vi "String To Number(I64)_csm.vi"(5 "String":string) -> (0 "Numeric(I64)":u64)   [LabVIEW 2017, in "API String Arguments Support.lvlib"]
uses:
  API String Arguments Support.lvlib
  35e04dae-fb20-45f2-b6e6-a1e99b0bae27.vi
  c7c8f582-3164-4c23-83d8-8f64db7f198b.vi
  <userlib>/_NEVSTOP/Communicable State Machine(CSM)/Communicable State Machine.lvlib
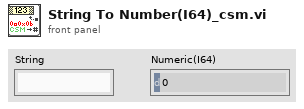
[diagram p1: front panel]
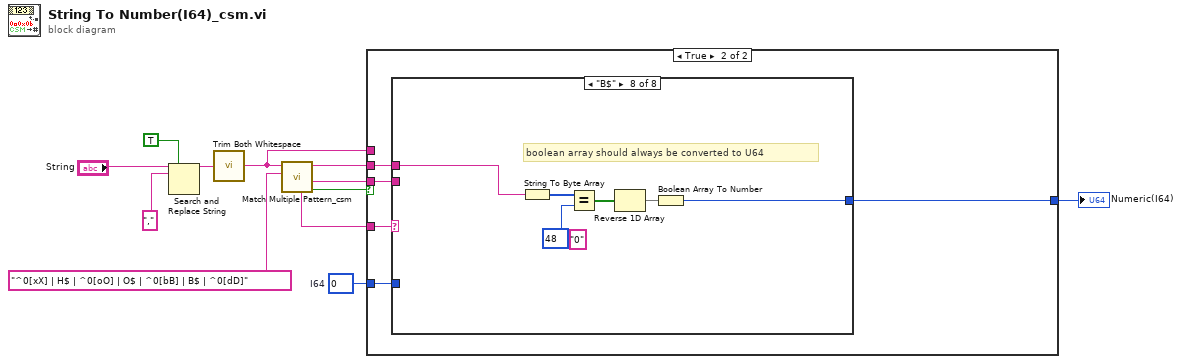
[diagram p0: block diagram]
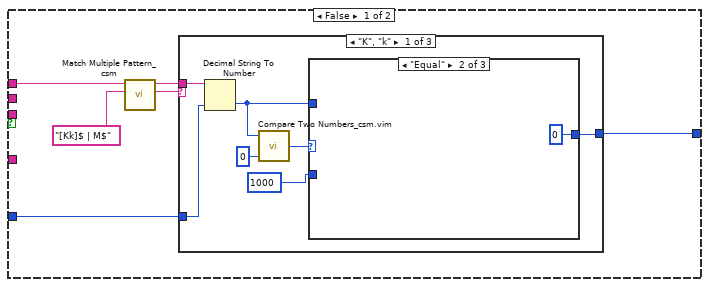
[diagram p2: hidden frame]
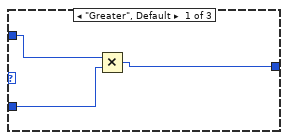
[diagram p3: hidden frame]
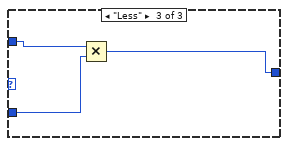
[diagram p4: hidden frame]
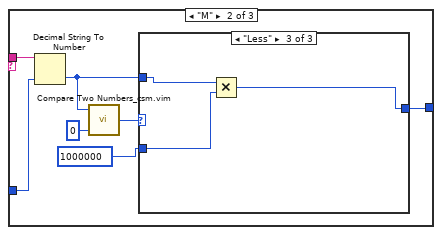
[diagram p5: hidden frame]
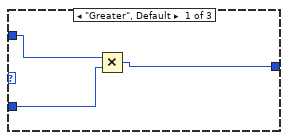
[diagram p6: hidden frame]
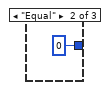
[diagram p7: hidden frame]
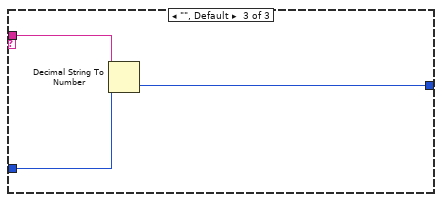
[diagram p8: hidden frame]
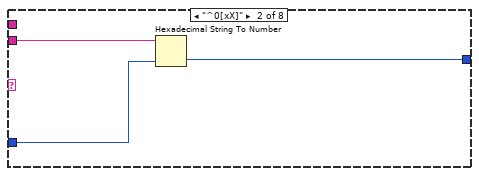
[diagram p10: hidden frame]
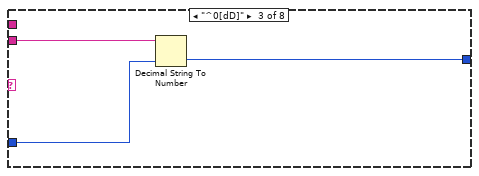
[diagram p11: hidden frame]
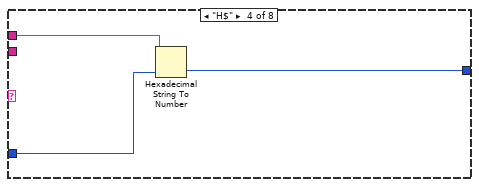
[diagram p12: hidden frame]
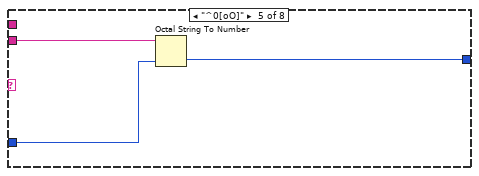
[diagram p13: hidden frame]
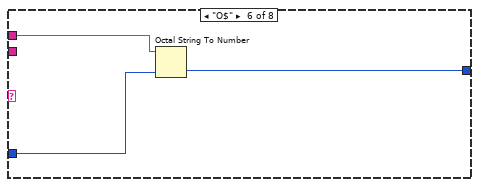
[diagram p14: hidden frame]
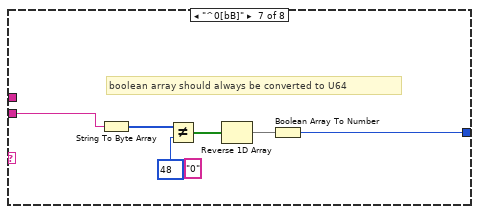
[diagram p15: hidden frame]
diagram:
  w1 = i64 0  # I64
  n1 = Search and Replace String(replace all?=TRUE ("replace all? (F)"), input string="String", search string=",") -> (result string=w9:string)  [unwired: 5 in, 3 out]
  n2 = call <userlib>:"Trim Both Whitespace.vi"("string"=w9) -> ("trimmed string"=w2:string)  [unwired: 1 in]
  n3 = call "Match Multiple Pattern_csm.vi"("regular expression"="^0[xX] | H$ | ^0[oO] | O$ | ^0[bB] | B$ | ^0[dD]", "string"=w2) -> ("Found?"=w7:bool, "after substring"=w5:string, "before substring"=w4:string, "pattern matched"=w6:string)  [unwired: 5 in, 1 out]
  n4 = case shown="True" w7 {
    tunnel: w6 -> [_ w54]
    tunnel: w5 -> [_ w53]
    tunnel: w4 -> [_ w52]
    tunnel: [w13 w51] -> w3
    tunnel: w2 -> [w14 _]
    tunnel: w1 -> [w15 w50]
    frame False {
      n5 = call "Match Multiple Pattern_csm.vi"("regular expression"="[Kk]$ | M$", "string"=w14) -> ("match substring"=w17:string, "before substring"=w16:string)  [unwired: 5 in, 3 out]
      n6 = case shown="\"K\", \"k\"" w17 {
        tunnel: [w22 w36 w49] -> w13
        tunnel: w15 -> [w21 w35 w48]
        tunnel: w16 -> [w25 w39 w47]
        frame "K", "k" {
          n7 = Decimal String To Number(string=w25, default (0L)=w21) -> (number=w20:i64)  [unwired: 1 in, 1 out]
          n8 = call "Compare Two Numbers_csm.vim"("Ref"=0, "Number"=w20) -> ("Result"=w23:enum16{"Greater", "Equal", "Less"})  [unwired: 1 in, 2 out]
          n9 = case shown="\"Equal\"" w23 {
            tunnel: [w28 i64 0 w32] -> w22
            tunnel: w20 -> [w27 _ w31]
            tunnel: i64 1000 ("y") -> [w26 _ w30]
            frame "Greater", Default {
              n10 = Multiply(x=w27, y=w26) -> (x*y=w28:i64)
            }
            frame "Equal" {
            }
            frame "Less" {
              n11 = Multiply(x=w31, y=w30) -> (x*y=w32:i64)
            }
          }
        }
        frame "M" {
          n12 = Decimal String To Number(string=w39, default (0L)=w35) -> (number=w34:i64)  [unwired: 1 in, 1 out]
          n13 = call "Compare Two Numbers_csm.vim"("Ref"=0, "Number"=w34) -> ("Result"=w37:enum16{"Greater", "Equal", "Less"})  [unwired: 1 in, 2 out]
          n14 = case shown="\"Less\"" w37 {
            tunnel: [w42 i64 0 w46] -> w36
            tunnel: w34 -> [w41 _ w45]
            tunnel: i64 1000000 ("y") -> [w40 _ w44]
            frame "Greater", Default {
              n15 = Multiply(x=w41, y=w40) -> (x*y=w42:i64)
            }
            frame "Equal" {
            }
            frame "Less" {
              n16 = Multiply(x=w45, y=w44) -> (x*y=w46:i64)
            }
          }
        }
        frame "", Default {
          n17 = Decimal String To Number(string=w47, default (0L)=w48) -> (number=w49:i64)  [unwired: 1 in, 1 out]
        }
      }
    }
    frame True {
      n18 = case shown="\"B$\"" w54 {
        tunnel: w53 -> [_ w58 w61 _ w67 _ w75 _]
        tunnel: w52 -> [_ _ _ w63 _ w69 _ w79]
        tunnel: [w55 w57 w60 w64 w66 w70 w76 w82] -> w51
        tunnel: w50 -> [w55 w56 w59 w62 w65 w68 _ _]
        frame Default {
        }
        frame "^0[xX]" {
          n19 = Hexadecimal String To Number(string=w58, default (0uL)=w56) -> (number=w57:i64)  [unwired: 1 in, 1 out]
        }
        frame "^0[dD]" {
          n20 = Decimal String To Number(string=w61, default (0L)=w59) -> (number=w60:i64)  [unwired: 1 in, 1 out]
        }
        frame "H$" {
          n21 = Hexadecimal String To Number(string=w63, default (0uL)=w62) -> (number=w64:i64)  [unwired: 1 in, 1 out]
        }
        frame "^0[oO]" {
          n22 = Octal String To Number(2:w65, 4:w67) -> (0:w66:i64)  [unwired: 1 in, 1 out]
        }
        frame "O$" {
          n23 = Octal String To Number(2:w68, 4:w69) -> (0:w70:i64)  [unwired: 1 in, 1 out]
        }
        frame "^0[bB]" {
          (unwired) "0" ("search string")
          # "boolean array should always be converted to U64"
          n24 = String To Byte Array(string=w75) -> (unsigned byte array=w74:u8[])
          n25 = Not Equal?(x=w74, y=u8 48) -> (x != y?=w72:bool[])
          n26 = Reverse 1D Array(array=w72) -> (reversed array=w71:bool[])
          n27 = Boolean Array To Number(Boolean array=w71) -> (number=w76:u64)
        }
        frame "B$" {
          (unwired) "0" ("search string")
          # "boolean array should always be converted to U64"
          n28 = String To Byte Array(string=w79) -> (unsigned byte array=w81:u8[])
          n29 = Equal?(x=w81, y=u8 48) -> (x = y?=w80:bool[])
          n30 = Reverse 1D Array(array=w80) -> (reversed array=w78:bool[])
          n31 = Boolean Array To Number(Boolean array=w78) -> (number=w82:u64)
        }
      }
    }
  }
  "Numeric(I64)" <- w3
